vi "Configure VIs.Progress Window.vi"(9 "Stop":refnum<data-value>, 10 "Progress":refnum<data-value>, 11 "Status String":refnum<data-value>) -> ()   [LabVIEW 2017]
panel:
  out "Status Message":string
  out "Progress":dbl(slide) scale=0.0..1.0 scale format="%.1f"
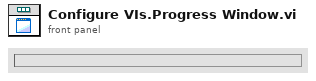
[diagram p1: front panel]
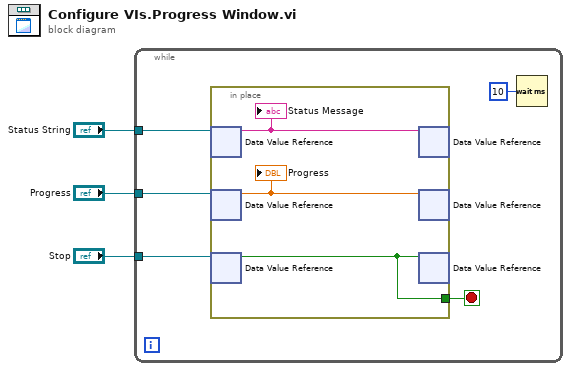
[diagram p0: block diagram]
diagram:
  n1 = while {
    tunnel: "Status String" -> [w7]
    tunnel: "Stop" -> [w6]
    tunnel: "Progress" -> [w4]
    stop <- w5 stop-if-true
    n2 = in-place {
      in-place-border: [w10] -> w5
      n3 = in-place-dvr #1(w7) -> (w11:string)  [unwired: 1 out]
      "Status Message" <- w11
      n4 = in-place-dvr #2(w4) -> (w9:dbl)  [unwired: 1 out]
      "Progress" <- w9
      n5 = in-place-dvr #3(w6) -> (w10:bool)  [unwired: 1 out]
      n6 = in-place-dvr #1(w11) -> ()  [unwired: 2 out]
      n7 = in-place-dvr #2(w9) -> ()  [unwired: 2 out]
      n8 = in-place-dvr #3(w10) -> ()  [unwired: 2 out]
    }
    n9 = Wait (ms)(milliseconds to wait=u32 10) -> ()  [unwired: 1 out]
  }
